vi "Intake.vi"   [LabVIEW 2017]
uses:
  <userlib>/836-Library/System/QCP_V2/QCPSupportCode/QCPData.ctl
  <userlib>/836-Library/System/QCP_V2/QCPSupportCode/QCP_GetDbl.vi
types:
  T1 = typedef "Semaphore RefNum" = refnum<k1>
  T2 = cluster{"Data Value Refnum":refnum<data-value>, "semaphore":T1}
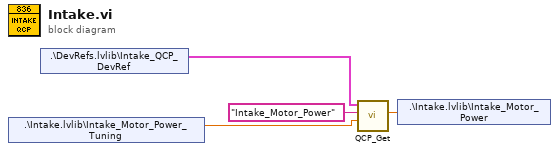
[diagram p0: block diagram]
diagram:
  n1 = shared-variable ".\\Intake.lvlib\\Intake_Motor_Power_Tuning"() -> (w2:dbl)  [unwired: 1 in, 1 out]
  n2 = shared-variable ".\\DevRefs.lvlib\\Intake_QCP_DevRef"() -> (w1:T2)  [unwired: 1 in, 1 out]
  n3 = call-poly <userlib>:"QCP_Get.vi"("Tuning Value"=w2, "Value Name"="Intake_Motor_Power", "QCP_DevRef_In"=w1) -> ("Value"=w4:dbl)  [unwired: 6 in, 2 out]
  n4 = shared-variable ".\\Intake.lvlib\\Intake_Motor_Power"(w4) -> ()  [unwired: 1 in, 1 out]
